vi "Positon Close Button.vi"(8 "error in (no error)":errorcluster, 11 "Button Ref":refnum<vi>) -> (0 "Error Out":errorcluster)   [LabVIEW 2014]
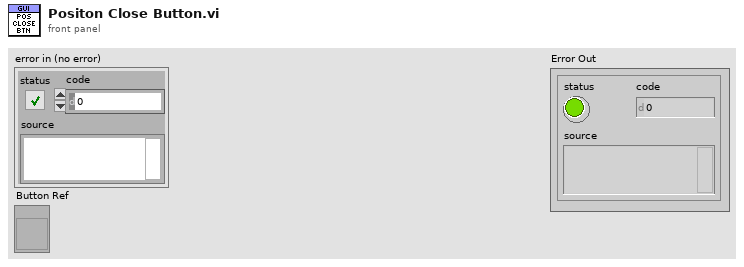
[diagram p1: front panel]
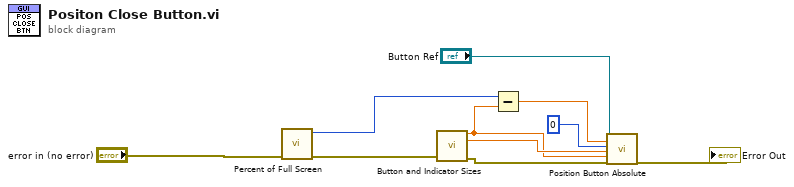
[diagram p0: block diagram]
diagram:
  n1 = call "Percent of Full Screen.vi"("error in (no error)"="error in (no error)") -> ("error out"=w9:errorcluster, "Right"=w8:i16)  [unwired: 8 in, 1 out]
  n2 = call "Button and Indicator Sizes.vi"("error in (no error)"=w9) -> ("Button Width"=w3:dbl, "Button Height"=w4:dbl, "error out"=w2:errorcluster)  [unwired: 10 in, 2 out]
  n3 = Subtract(x=w8, y=w3) -> (x-y=w7:dbl)
  n4 = call "Position Button Absolute.vi"("Button Ref"="Button Ref", "Left Offset (px)"=w7, "Top Offste (px)"=0, "Height (px)"=w4, "Width (px)"=w3, "Error In"=w2) -> ("Error Out"=→"Error Out":errorcluster)  [unwired: 13 in]
